vi "Module Init.vi"(8 "error in (no error)":errorcluster, 11 "Volatus Core in":refnum<class "Volatus Core.lvclass">) -> (0 "error out":errorcluster, 3 "Volatus Core out":refnum<class "Volatus Core.lvclass">)   [LabVIEW 2020, in "Volatus.lvlib" / "Volatus Core.lvclass"]
uses:
  Volatus Core.lvclass
  C:/dev/lv20CE/relink/lv-volatus/Volatus/Module/Module.lvclass
  Module/Module.lvclass/Module.ctl
  Volatus Core.lvclass/Volatus Core.ctl
  Volatus.lvlib
  Module/Module.lvclass
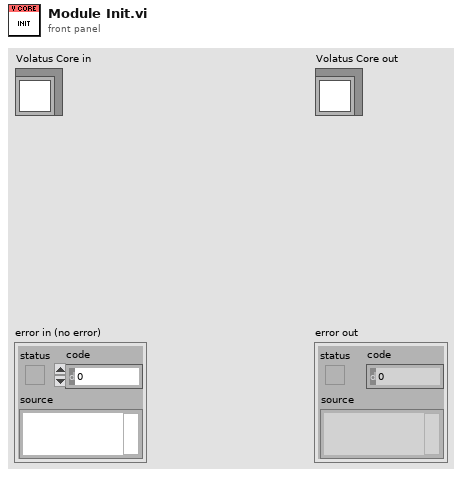
[diagram p1: front panel]
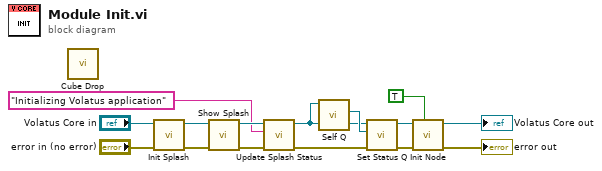
[diagram p0: block diagram]
diagram:
  n1 = call "Cube Drop.vi"() -> ()  [unwired: 12 in]
  n2 = call "Init Splash.vi"("error in (no error)"="error in (no error)", "Volatus Core in"="Volatus Core in") -> ("error out"=w3:errorcluster, "Volatus Core out"=w1:refnum<class "Volatus Core.lvclass">)  [unwired: 8 in]
  n3 = call "Show Splash.vi"("error in (no error)"=w3, "Volatus Core in"=w1) -> ("error out"=w8:errorcluster, "Volatus Core out"=w6:refnum<class "Volatus Core.lvclass">)  [unwired: 8 in]
  n4 = call "Update Splash Status.vi"("error in (no error)"=w8, "Status"="Initializing Volatus application", "Volatus Core in"=w6) -> ("error out"=w7:errorcluster, "Volatus Core out"=w5:refnum<class "Volatus Core.lvclass">)  [unwired: 7 in]
  n5 = call "Self Q.vi"("Module in"=w5) -> ("Self Q"=w9:refnum<class "MessageQ.lvclass">)  [unwired: 9 in, 1 out]
  n6 = call "Set Status Q.vi"("error in (no error)"=w7, "Status Q"=w9, "Module in"=w5) -> ("error out"=w11:errorcluster, "Module out"=w10:refnum<class "Volatus Core.lvclass">)  [unwired: 7 in]
  n7 = call "Init Node.vi"("First Launch"=TRUE ("Launch Events"), "error in (no error)"=w11, "Volatus Core in"=w10) -> ("error out"=→"error out":errorcluster, "Volatus Core out"=→"Volatus Core out":refnum<class "Volatus Core.lvclass">)  [unwired: 7 in]
